vi "Sort name chrono.vi"(4 "Names":string[](array[string])) -> (1 "Names Sorted":string[](array[string]))   [LabVIEW 2009]
uses:
  <vilib>/regexp/Match Regular Expression.xnode
panel:
  # "Guillaume Plateau - yguig2@yahoo.fr"
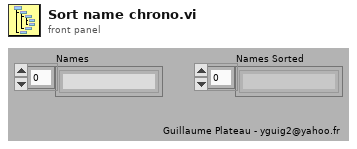
[diagram p1: front panel]
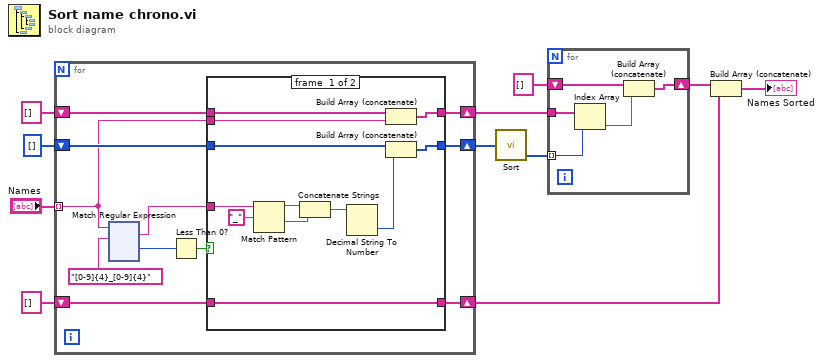
[diagram p0: block diagram]
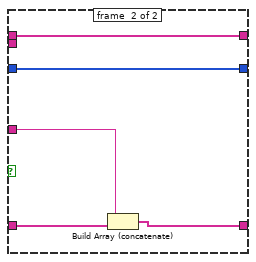
[diagram p2: hidden frame]
diagram:
  n1 = for {
    tunnel: "Names" -> [w13] mode=indexing
    shift-right: [w20] -> w2
    shift-left: string[] [] -> [w21]
    shift-right: [w15] -> w4
    shift-left: string[] [] -> [w16]
    shift-right: [w18] -> w7
    shift-left: i32[] [] -> [w19]
    n2 = xnode "Match Regular Expression"("input string"=w13, "regular expression"="[0-9]{4}_[0-9]{4}") -> ("whole match"=w17:string, "offset past match"=w12:i32)  [unwired: 4 in, 3 out]
    n3 = Less Than 0?(x=w12) -> (x < 0?=w22:bool)
    n4 = case shown="False" w22 {
      tunnel: w17 -> [w140 w146]
      tunnel: w21 -> [w141 w145]
      tunnel: [w141 w144] -> w20
      tunnel: w19 -> [w135 w142]
      tunnel: [w133 w142] -> w18
      tunnel: w16 -> [w132 w143]
      tunnel: w13 -> [w131 _]
      tunnel: [w130 w143] -> w15
      frame #0 {
        n5 = Match Pattern(string=w140, regular expression="_" ("search string/char (-)")) -> (before substring=w138:string, after substring=w137:string)  [unwired: 1 in, 2 out]
        n6 = Concatenate Strings(w138, w137) -> (w136:string)
        n7 = Decimal String To Number(string=w136) -> (number=w134:i32)  [unwired: 2 in, 1 out]
        n8 = Build Array (concatenate)(w132, w131) -> (w130:string[])
        n9 = Build Array (concatenate)(w135, w134) -> (w133:i32[])
      }
      frame #1 {
        n10 = Build Array (concatenate)(w146, w145) -> (w144:string[])
      }
    }
  }
  n11 = call "Sort.vi"("Array"=w7) -> ("Indices"=w5:i32[])  [unwired: 3 in, 1 out]
  n12 = for {
    shift-right: [w147] -> w3
    shift-left: string[] [] -> [w149]
    tunnel: w5 -> [w150] mode=indexing
    tunnel: w4 -> [w151]
    n13 = Index Array(array=w151, index=w150) -> (element=w148:string)
    n14 = Build Array (concatenate)(w149, w148) -> (w147:string[])
  }
  n15 = Build Array (concatenate)(w3, w2) -> (→"Names Sorted":string[])
